vi "SWITCH Configure.vi"(8 "error in (no error)":errorcluster, 10 "Message Data":variant, 11 "Data Cluster":T1={"Tango HW"={"VISA resource"="", "Baud Rate (115200)"=2, "lAnInterfaceType"=0, "bAShowProt"=15}, "Writer Queue"=refnum, "Status"=FALSE, "Abs Position"=[], "Axis Velocity"={"dX"=0.0, "dY"=0.0, "dZ"=0.0, "dA"=0.0}, "acceleration "=0.0, "Z direction"=enum."Up", "Position Mode"="", "plLSID"=0}) -> (0 "error out":errorcluster, 2 "Send Resp":bool, 3 "Data Cluster out":T1={"Tango HW"={"VISA resource"="", "Baud Rate (115200)"=2, "lAnInterfaceType"=0, "bAShowProt"=15}, "Writer Queue"=refnum, "Status"=FALSE, "Abs Position"=[], "Axis Velocity"={"dX"=0.0, "dY"=0.0, "dZ"=0.0, "dA"=0.0}, "acceleration "=0.0, "Z direction"=enum."Up", "Position Mode"="", "plLSID"=0})   [LabVIEW 2020, in "MOTOR.lvlib"]
uses:
  MOTOR.lvlib
  PS Hardware Configuration.ctl
  support/Message Queue/Message Cluster.ctl
  support/Message Queue/Message Queue.lvlib
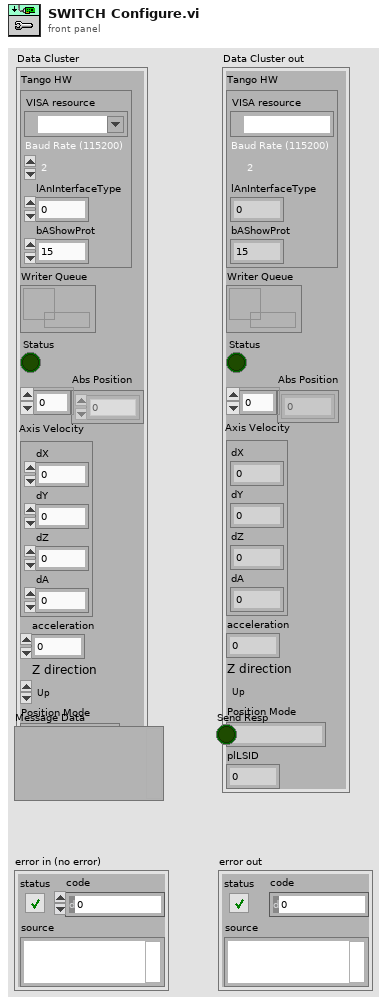
[diagram p1: front panel]
types:
  T1 = typedef "MOTOR.lvlib/PS Hardware Configuration.ctl" = cluster{"Tango HW":cluster{"VISA resource":refnum<visa-resource-name>, "Baud Rate (115200)":i32, "lAnInterfaceType":i32, "bAShowProt":i32}, "Writer Queue":refnum<queue>, "Status":bool, "Abs Position":i32[], "Axis Velocity":cluster{"dX":dbl, "dY":dbl, "dZ":dbl, "dA":dbl}, "acceleration ":dbl, "Z direction":enum16{"Up", "Down"}, "Position Mode":string, "plLSID":i32}
  T2 = typedef "Message Queue.lvlib/Message Cluster.ctl" = cluster{"Message":string, "Message Data":variant}
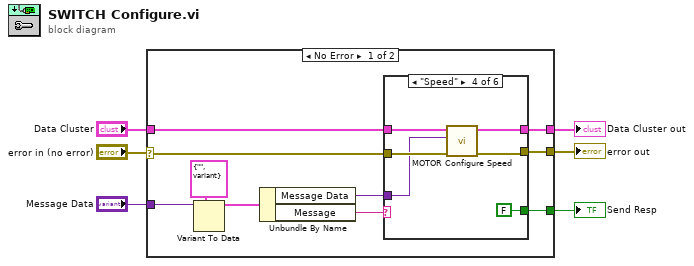
[diagram p0: block diagram]
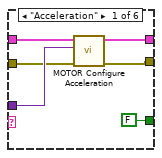
[diagram p2: hidden frame]
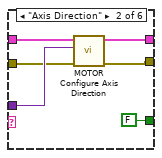
[diagram p3: hidden frame]
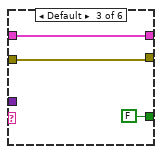
[diagram p4: hidden frame]
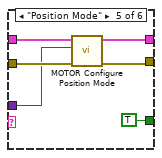
[diagram p5: hidden frame]
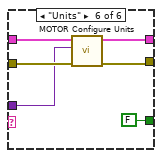
[diagram p6: hidden frame]
diagram:
  n1 = case shown="No Error" "error in (no error)" {
    selector: "error in (no error)" -> [w9 w50]
    tunnel: [w16 w50] -> w6
    tunnel: "Data Cluster" -> [w15 w51]
    tunnel: [w14 w51] -> w4
    tunnel: "Message Data" -> [w10 _]
    tunnel: [w7 _] -> w1
    frame No Error {
      n2 = Variant To Data(type=T2 {"Message"="", "Message Data"=variant} ("element"), Variant=w10) -> (data=w12:T2)  [unwired: 1 in, 1 out]
      n3 = Unbundle By Name(w12) -> ("Message Data"=w8:variant, "Message"=w13:string)
      n4 = case shown="\"Speed\"" w13 {
        tunnel: w8 -> [w19 w25 _ w33 w39 w45]
        tunnel: [w20 w26 w30 w35 w41 w47] -> w14
        tunnel: w15 -> [w21 w27 w30 w36 w42 w48]
        tunnel: w9 -> [w18 w24 w29 w34 w40 w46]
        tunnel: [w17 w23 w29 w32 w38 w44] -> w16
        tunnel: [FALSE ("Send Resp") FALSE ("Send Resp") FALSE ("Send Resp") FALSE ("Send Resp") TRUE ("Send Resp") FALSE ("Send Resp")] -> w7
        frame "Acceleration" {
          n5 = call "MOTOR Configure Acceleration.vi"("error in (no error)"=w18, "Message Data"=w19, "Data Cluster in"=w21) -> ("error out"=w17:errorcluster, "Data Cluster out"=w20:T1)  [unwired: 7 in]
        }
        frame "Axis Direction" {
          n6 = call "MOTOR Configure Axis Direction.vi"("error in (no error)"=w24, "Message Data"=w25, "Data Cluster in"=w27) -> ("error out"=w23:errorcluster, "Data Cluster out"=w26:T1)  [unwired: 7 in]
        }
        frame Default {
        }
        frame "Speed" {
          n7 = call "MOTOR Configure Speed.vi"("error in (no error)"=w34, "Message Data"=w33, "Data Cluster in"=w36) -> ("error out"=w32:errorcluster, "Data Cluster out"=w35:T1)  [unwired: 7 in]
        }
        frame "Position Mode" {
          n8 = call "MOTOR Configure Position Mode.vi"("error in (no error)"=w40, "Message Data"=w39, "Data Cluster in"=w42) -> ("error out"=w38:errorcluster, "Data Cluster out"=w41:T1)  [unwired: 7 in]
        }
        frame "Units" {
          n9 = call "MOTOR Configure Units.vi"("error in (no error)"=w46, "Message Data"=w45, "Data Cluster in"=w48) -> ("error out"=w44:errorcluster, "Data Cluster out"=w47:T1)  [unwired: 7 in]
        }
      }
    }
    frame Error {
    }
  }
  "error out" <- w6
  "Data Cluster out" <- w4
  "Send Resp" <- w1
